vi "Launch Nested Actors.vi"(8 "error in (no error)":errorcluster, 11 "ATM Controller in":refnum<class "ATM Controller.lvclass">) -> (0 "error out":errorcluster, 3 "ATM Controller out":refnum<class "ATM Controller.lvclass">)   [LabVIEW 2019, in "ATM Controller.lvlib" / "ATM Controller.lvclass"]
uses:
  ATM Controller.lvclass
  C:/Program Files (x86)/National Instruments/LabVIEW 2019/vi.lib/ActorFramework/Actor/Actor.lvclass
  Sim User Console Actor/ATM Controller/Sim User Console Actor.lvclass
  Sim Display Console Actor/ATM Controller/Sim Display Console Actor.lvclass
  Sim Sensor Interface Actor/ATM Controller/Sim Sensor Interface Actor.lvclass
  Configuration Database/Configuration Database/Configuration Database.lvclass
  ATM Controller.lvclass/ATM Controller.ctl
  <vilib>/ActorFramework/Actor/Actor.lvclass
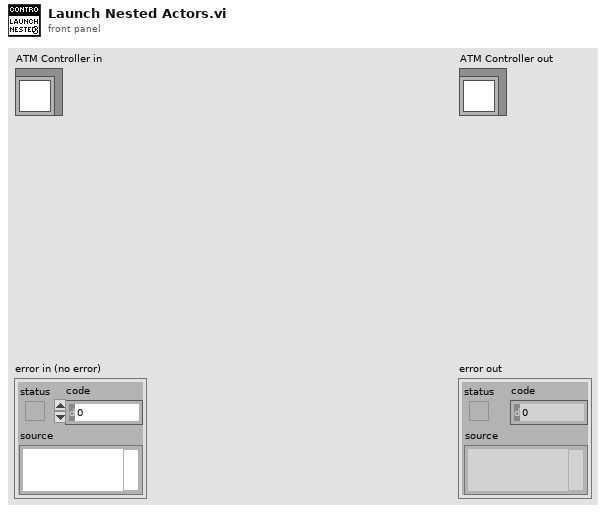
[diagram p1: front panel]
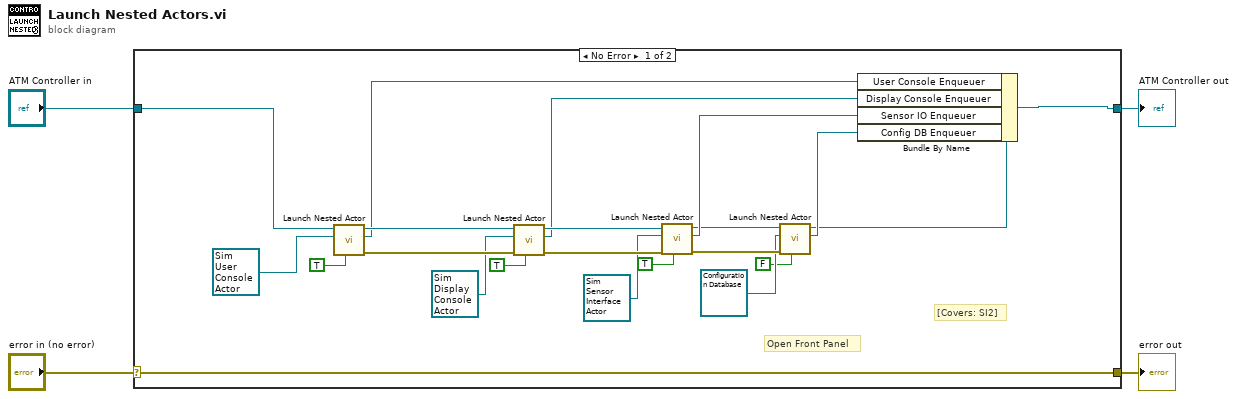
[diagram p0: block diagram]
diagram:
  n1 = case shown="No Error" "error in (no error)" {
    selector: "error in (no error)" -> [w26 w28]
    tunnel: [w26 w28] -> w3
    tunnel: [w19 w27] -> w1
    tunnel: "ATM Controller in" -> [w14 w27]
    frame No Error {
      # "[Covers: SI2]"
      # "Open Front Panel"
      n2 = call <vilib>:"Launch Nested Actor.vi"("Open Actor Core front panel? (F)"=TRUE, "Nested Actor"=refnum<class "Sim User Console Actor.lvclass"> refnum ("Sim User Console Actor.lvlib:Sim User Console Actor.lvclass"), "Caller Actor in"=w14) -> ("error out"=w22:errorcluster, "Nested Actor's Enqueuer"=w13:refnum<class "Message Enqueuer.lvclass">, "Caller Actor out"=w23:refnum<class "ATM Controller.lvclass">)  [unwired: 6 in]
      n3 = call <vilib>:"Launch Nested Actor.vi"("Open Actor Core front panel? (F)"=TRUE, "error in (no error)"=w22, "Nested Actor"=refnum<class "Sim Display Console Actor.lvclass"> refnum ("Sim Display Console Actor.lvlib:Sim Display Console Actor.lvclass"), "Caller Actor in"=w23) -> ("error out"=w17:errorcluster, "Nested Actor's Enqueuer"=w12:refnum<class "Message Enqueuer.lvclass">, "Caller Actor out"=w18:refnum<class "ATM Controller.lvclass">)  [unwired: 5 in]
      n4 = call <vilib>:"Launch Nested Actor.vi"("Open Actor Core front panel? (F)"=TRUE, "error in (no error)"=w17, "Nested Actor"=refnum<class "Sim Sensor Interface Actor.lvclass"> refnum ("Sim Sensor Interface Actor.lvlib:Sim Sensor Interface Actor.lvclass"), "Caller Actor in"=w18) -> ("error out"=w9:errorcluster, "Nested Actor's Enqueuer"=w11:refnum<class "Message Enqueuer.lvclass">, "Caller Actor out"=w10:refnum<class "ATM Controller.lvclass">)  [unwired: 5 in]
      n5 = call <vilib>:"Launch Nested Actor.vi"("Open Actor Core front panel? (F)"=FALSE, "error in (no error)"=w9, "Nested Actor"=refnum<class "Configuration Database.lvclass"> refnum ("Configuration Database.lvlib:Configuration Database.lvclass"), "Caller Actor in"=w10) -> ("Nested Actor's Enqueuer"=w8:refnum<class "Message Enqueuer.lvclass">, "Caller Actor out"=w5:refnum<class "ATM Controller.lvclass">)  [unwired: 5 in, 1 out]
      n6 = Bundle By Name(cluster=w5, "User Console Enqueuer"=w13, "Display Console Enqueuer"=w12, "Sensor IO Enqueuer"=w11, "Config DB Enqueuer"=w8) -> (w19:refnum<class "ATM Controller.lvclass">)
    }
    frame Error {
    }
  }
  "error out" <- w3
  "ATM Controller out" <- w1
